vi "RT Loop - Analyze Acceleration_queue_1.vi"(7 "testing":bool, 8 "error in (no error)":errorcluster, 9 "Acceleration RT FIFO In":T1, 10 "FPGA VI Reference Out":refnum<k20>, 11 "Message Queue":refnum<queue>) -> (1 "Acceleration RT FIFO Out":T1)   [LabVIEW 2017]
doc: "Read and analyze acceleration waveform data from FPGA via DMA FIFO. If the acceleration is over the limit, then send the acceleration waveform data to the Log Data Loop."
uses:
  <vilib>/rvi/interface/nirviMethod/nirviMethod.xnode
  <vilib>/FPGAPlugInAG/Dynamic/niLvFpga_ReadFifo_Dynamic.vi
  <vilib>/rvi/errors/niLvFpgaMergeErrorWithErrorCode.vi
  Globals/Global - All RT Loop Stop.vi
  Globals/Global - Configuration Options.vi
  UI Error Handlers/support/Logging/Logging.lvlib
  UI Error Handlers/support/Message Queue/Message Cluster.ctl
  UI Error Handlers/support/Message Queue/Message Queue.lvlib
  controls/Acceleration RT FIFO Reference.ctl
panel:
  out "AVI Path 2":path
  out "G1 status.G1 trigger 3":bool
  out "error out 3":errorcluster
  out "error out 2":errorcluster
  out "AVI Path":path
  out "G1 status.G1 trigger 2":bool
  out "error out":errorcluster
  out "Array":waveform(dbl)[](array[waveform])
  out "x-y":u32
  out "G1 status":cluster{"G1 trigger":bool}
  out "G1 status.G1 trigger":bool
  out "sta":bool
  out "logical OR":bool
  in  "Data Rate (Hz)":dbl
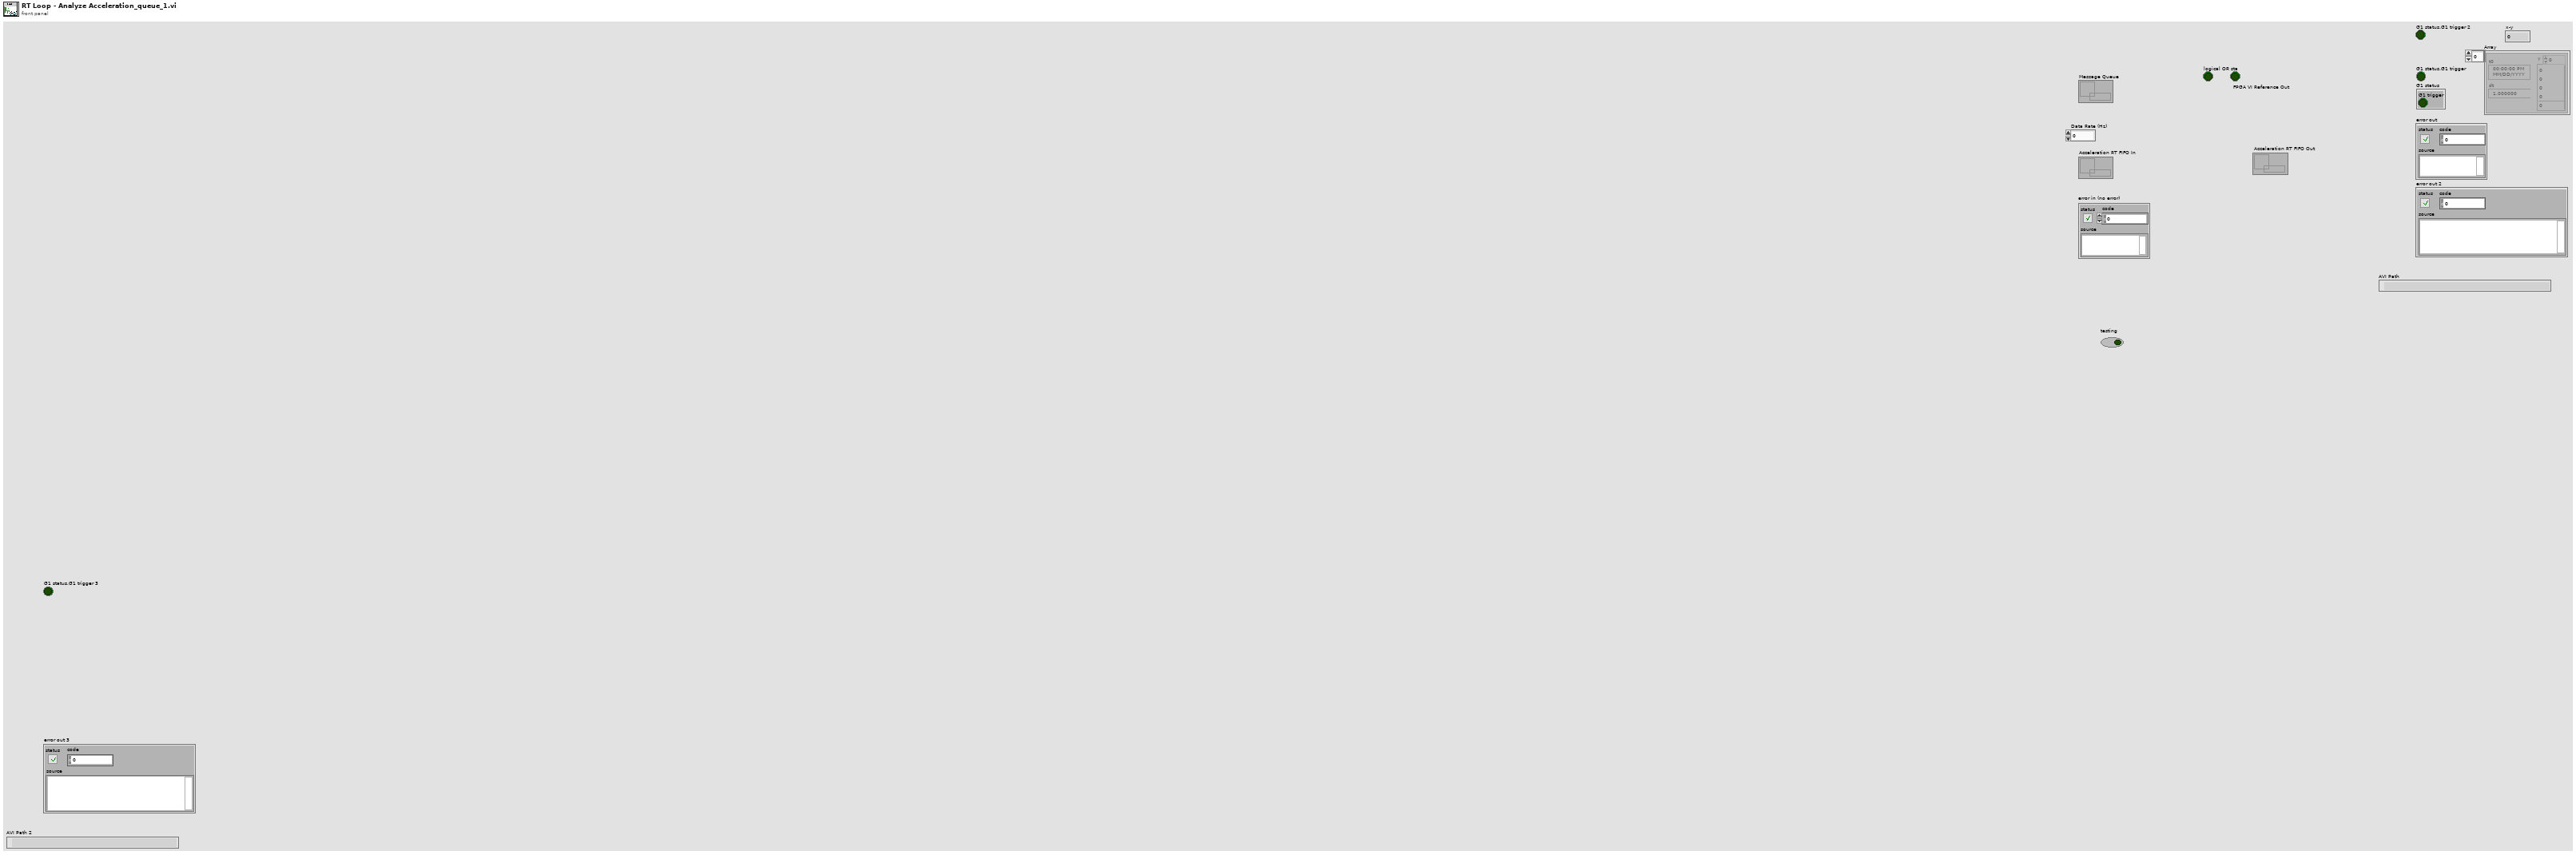
[diagram p1: front panel]
types:
  T1 = typedef "Acceleration RT FIFO Reference.ctl" = refnum<k33>
  T2 = cluster{"Tool data":cluster{"Number of teeth":sgl}, "Cutting data":cluster{"rpm":sgl}, "Limits":cluster{"Magnitude threshold":sgl, "Tolerance":sgl}, "G1 status":cluster{"G1 trigger":bool}}
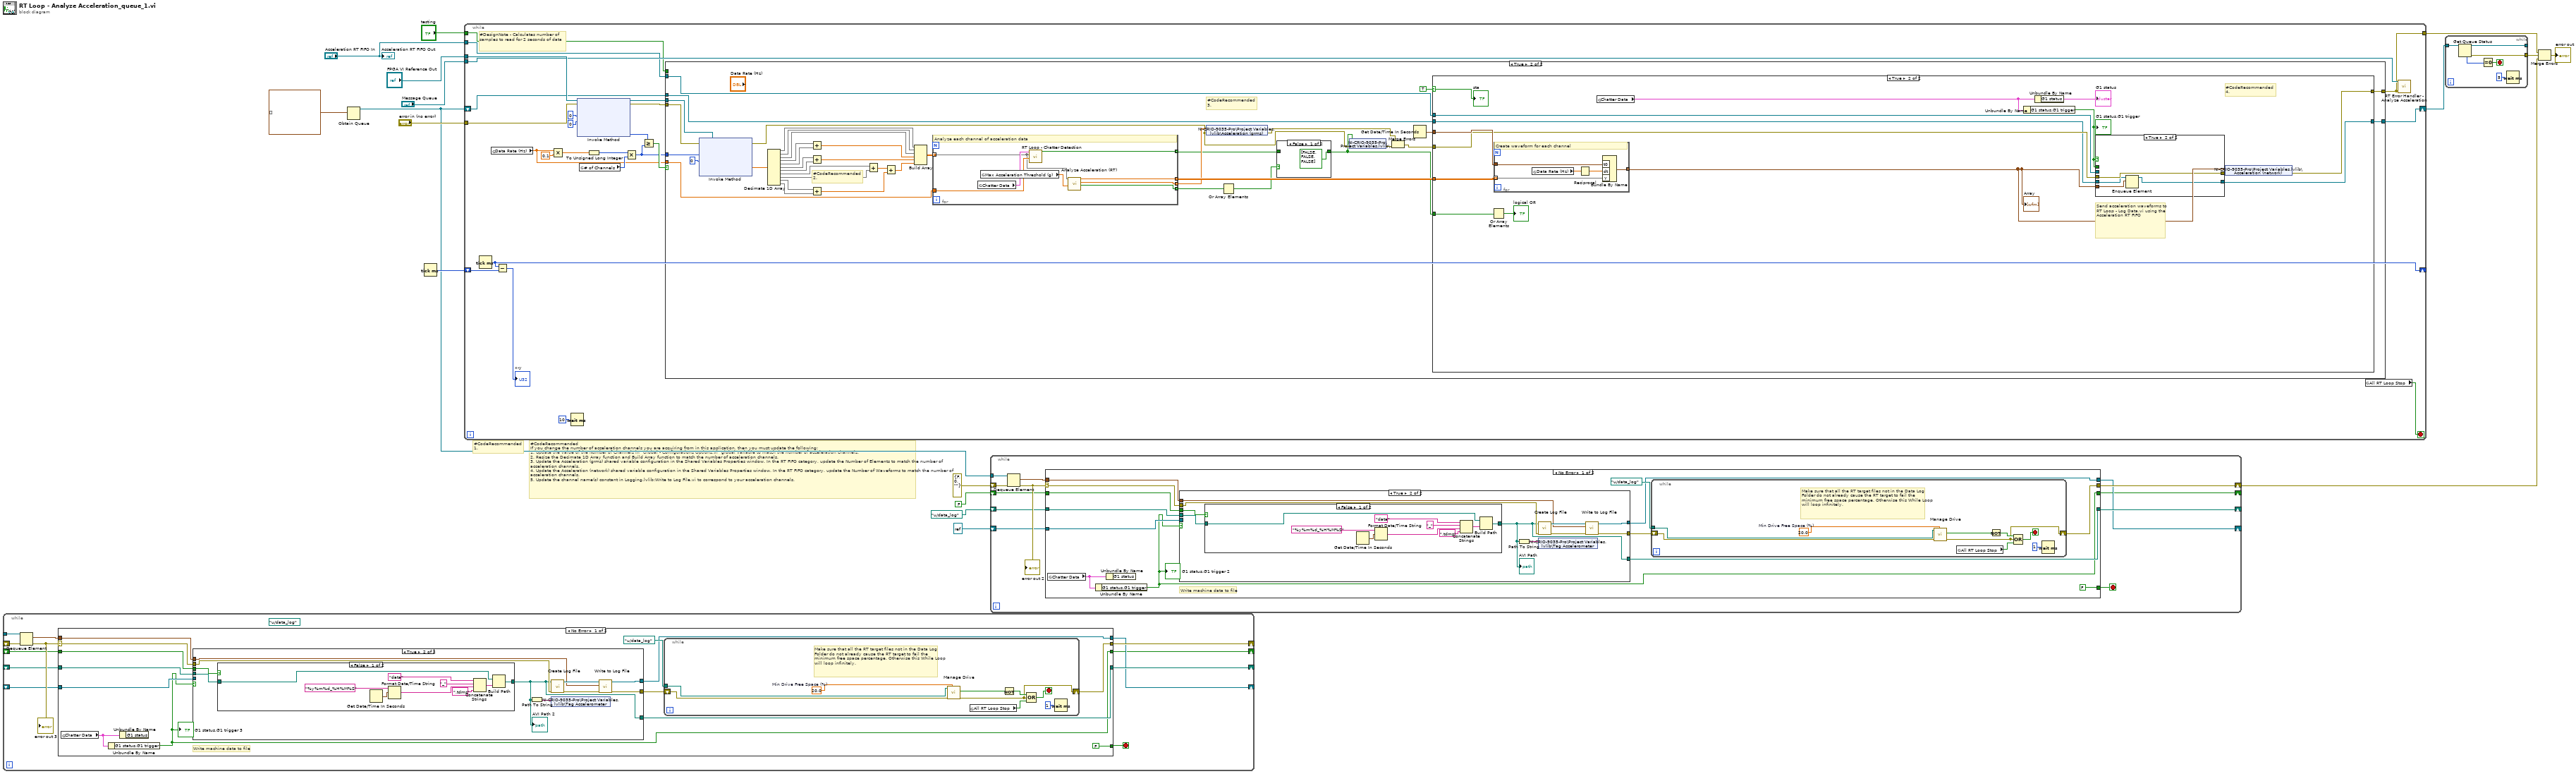
[diagram p0: block diagram]
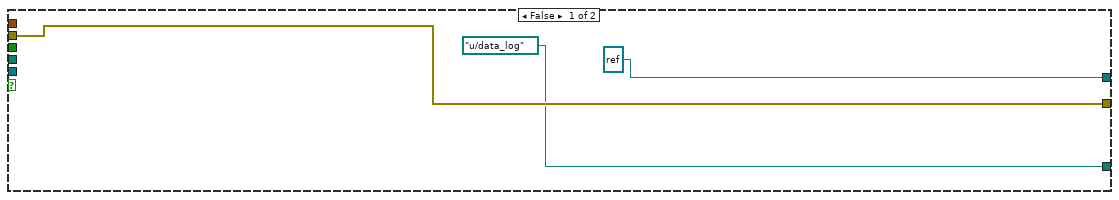
[diagram p2: hidden frame]
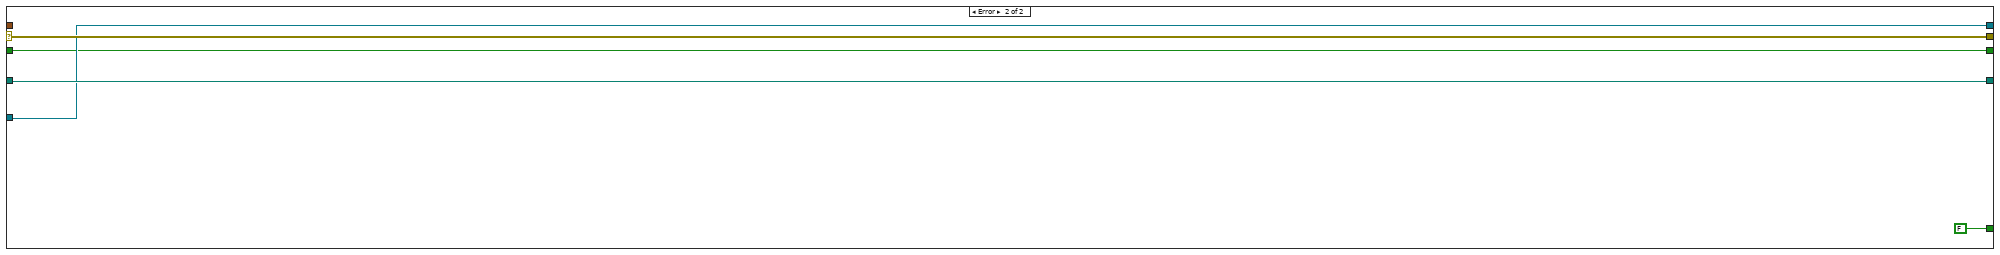
[diagram p4: hidden frame]
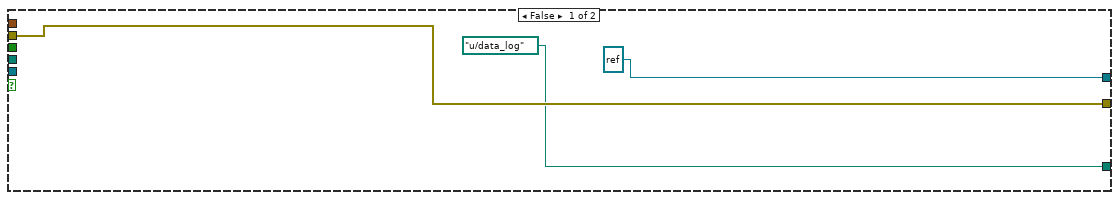
[diagram p5: hidden frame]
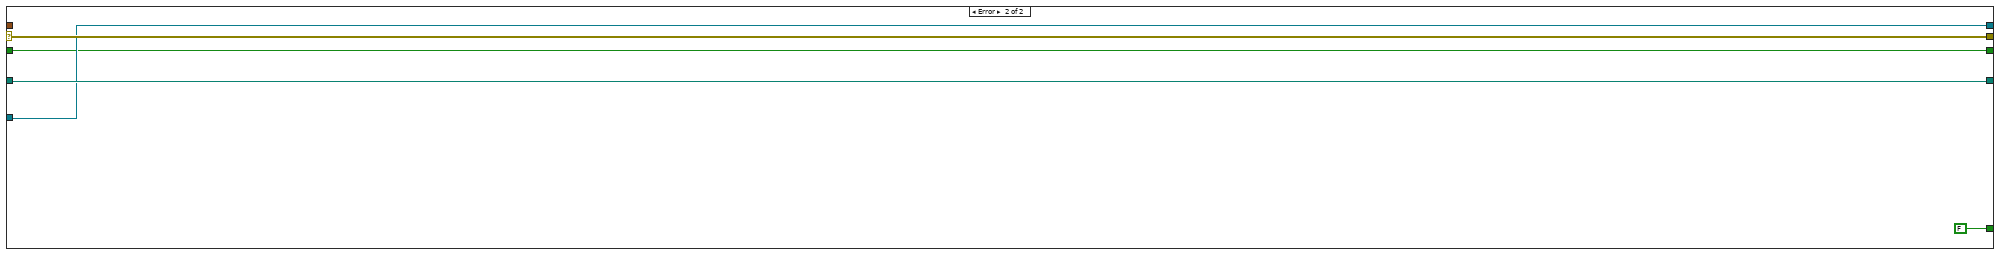
[diagram p7: hidden frame]
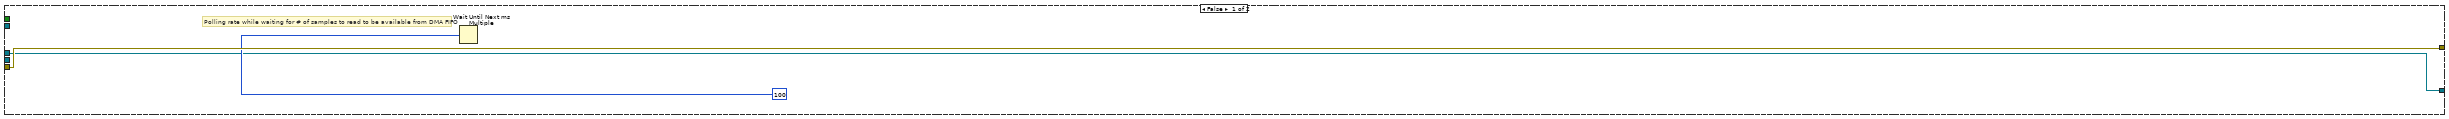
[diagram p8: hidden frame]
diagram:
  (unwired) path "u:/data_log" ("AVI Path")
  # "#CodeRecommended\n1."
  # "#CodeRecommended\nIf you change the number of acceleration channels you are acquiring from in this application, then you must update the following:\n1. Update the value of the Number of Channels in \"Global - Configurations Options.vi\" global variable to match the number of acceleration channels.\n2. Resize the Decimate 1D Array function and Build Array function to match the number of acceleration channels. \n3. Update the Acceleration (grms) shared variable configuration in the Shared Variables Properties window. In the RT FIFO category, update the Number of Elements to match the number of acceleration channels. \n4. Update the Acceleration (network) shared variable configuration in the Shared Variables Properties window. In the RT FIFO category, update the Number of Waveforms to match the number of acceleration channels.\n5. Update the channel name(s) constant in Logging.lvlib:Write to Log File.vi to correspond to your acceleration channels."
  n1 = while {
    tunnel: _ -> [w29]
    shift-right: [w25] -> _
    shift-left: _ -> [w28]
    shift-right: [w18] -> _
    shift-left: _ -> [w21]
    shift-right: [w23] -> _
    shift-left: _ -> [w24]
    shift-right: [w20] -> _
    shift-left: _ -> [w19]
    stop <- w26 stop-if-true
    n2 = Dequeue Element(queue=w29, error in (no error)=w28) -> (element=w22:waveform(dbl)[], error out=w27:errorcluster)  [unwired: 1 in, 2 out]
    "error out 3" <- w27
    n3 = case shown="No Error" w27 {
      selector: w27 -> [w37 w78]
      tunnel: [FALSE FALSE] -> w26
      tunnel: [w35 w78] -> w25
      tunnel: w24 -> [w41 w77]
      tunnel: [w40 w77] -> w23
      tunnel: w22 -> [w39 _]
      tunnel: w21 -> [w34 w75]
      tunnel: [w33 w76] -> w20
      tunnel: w19 -> [w32 w76]
      tunnel: [w30 w75] -> w18
      frame No Error {
        # "Write machine data to file"
        n4 = global read "Global - Configuration Options.vi" "Chatter Data"() -> (w31:T2)
        n5 = Unbundle By Name(w31) -> ("G1 status.G1 trigger"=w30:bool)
        "G1 status.G1 trigger 3" <- w30
        n6 = Unbundle By Name(w31) -> ()  [unwired: 1 out]
        n7 = case shown="True" w30 {
          tunnel: w41 -> [_ w64]
          tunnel: [path "u:/data_log" ("AVI Path") w56] -> w40
          tunnel: w39 -> [_ w60]
          tunnel: w37 -> [w54 w59]
          tunnel: [w54 w58] -> w36
          tunnel: w34 -> [_ w55]
          tunnel: [refnum<k34> refnum ("Log File out") w57] -> w33
          tunnel: w32 -> [_ _]
          frame False {
          }
          frame True {
            n8 = case shown="False" w55 {
              tunnel: w64 -> [w67 w74]
              tunnel: [w66 w74] -> w56
              frame False {
                n9 = Get Date/Time In Seconds() -> (seconds since 1Jan1904=w69:timestamp)
                n10 = Format Date/Time String(time format string (%c)="%y%m%d_%H%M%S", seconds (now)=w69) -> (date/time string=w72:string)  [unwired: 1 out]
                n11 = Concatenate Strings("data" ("string"), "_" ("string"), w72, ".tdms" ("string")) -> (w68:string)
                n12 = Build Path(base path=w67, name or relative path=w68) -> (appended path=w66:path)
              }
              frame True {
              }
            }
            "AVI Path 2" <- w56
            n13 = Path To String(path=w56) -> (string=w61:string)
            n14 = call "Create Log File.vi"("error in (no error)"=w59, "Acceleration Exceeded Log Folder"=w56) -> ("error out"=w63:errorcluster, "Log File out"=w62:refnum<k34>)  [unwired: 8 in]
            n15 = shared-variable "NI-CRIO-9035-Pro\\Project Variables.lvlib\\Tag Accelerometer"(w61) -> ()  [unwired: 1 in, 1 out]
            n16 = call "Write to Log File.vi"("error in (no error)"=w63, "Array of Waveforms"=w60, "Log File in"=w62) -> ("error out"=w58:errorcluster, "Log File out"=w57:refnum<k34>)  [unwired: 7 in]
          }
        }
        n17 = while {
          shift-right: [w46] -> w35
          shift-left: w36 -> [w47]
          tunnel: path "u:/data_log" ("AVI Path") -> [w44]
          stop <- w51 stop-if-true
          w45 = 20.0  # Min Drive Free Space (%)
          # "Make sure that all the RT target files not in the Data Log Folder do not already cause the RT target to fail the minimum free space percentage. Otherwise this While Loop will loop infinitely."
          n18 = call "Manage Drive.vi"("Min Drive Free Space (%)"=w45, "error in"=w47, "Data Folder"=w44) -> ("error out"=w46:errorcluster, "Drive Space Below Limit"=w43:bool)  [unwired: 7 in]
          n19 = global read "Global - All RT Loop Stop.vi" "All RT Loop Stop"() -> (w48:bool)
          n20 = Not(x=w43) -> (.not. x?=w50:bool)
          n21 = Compound Arithmetic op=OR(w50, w46, w48) -> (w51:bool)
          n22 = Wait (ms)(milliseconds to wait=u32 1) -> ()  [unwired: 1 out]
        }
      }
      frame Error {
      }
    }
  }
  n23 = Obtain Queue(element data type=waveform(dbl)[] [] ("Array 2")) -> (queue out=w5:refnum<queue>)  [unwired: 4 in, 2 out]
  n24 = Tick Count (ms)() -> (millisecond timer value=w12:u32)
  n25 = while {
    tunnel: "FPGA VI Reference Out" -> [w104]
    tunnel: "error in (no error)" -> [w103]
    tunnel: "Message Queue" -> [w96]
    tunnel: "Acceleration RT FIFO In" -> [w95]
    tunnel: "testing" -> [w87]
    shift-right: [w85] -> _
    shift-left: w12 -> [w86]
    shift-right: [w82] -> w4
    shift-left: w5 -> [w83]
    tunnel: [w81] -> w2
    stop <- w97 stop-if-true
    # "#DesignNote - Calculates number of samples to read for 2 seconds of data"
    n26 = Tick Count (ms)() -> (millisecond timer value=w85:u32)
    n27 = global read "Global - Configuration Options.vi" "Data Rate (Hz)"() -> (w89:dbl)
    n28 = Subtract(x=w85, y=w86) -> (x-y=→"x-y":u32)
    n29 = Multiply(x=w89, y=0.1) -> (x*y=w93:dbl)
    n30 = Wait (ms)(milliseconds to wait=u32 10) -> ()  [unwired: 1 out]
    n31 = xnode "Invoke Method"("FPGA VI Reference In"=w104, "error in"=w103, "Number of Elements"=u32 0, "Timeout (ms)"=0) -> ("FPGA VI Reference Out"=w100:refnum<k20>, "error out"=w99:errorcluster, "Elements Remaining"=w88:u32)  [unwired: 1 out]
    n32 = global read "Global - Configuration Options.vi" "# of Channels"() -> (w90:u32)
    n33 = To Unsigned Long Integer(number=w93) -> (unsigned 32bit integer=w92:u32)
    n34 = Multiply(x=w92, y=w90) -> (x*y=w91:u32)
    n35 = Greater Or Equal?(x=w88, y=w91) -> (x >= y?=w98:bool)
    n36 = case shown="True" w98 {
      tunnel: w100 -> [_ w146]
      tunnel: w99 -> [w107 w145]
      tunnel: [w107 w141] -> w81
      tunnel: w91 -> [_ w144]
      tunnel: w95 -> [_ w139]
      tunnel: w89 -> [_ w135]
      tunnel: w87 -> [_ _]
      tunnel: w83 -> [w105 w109]
      tunnel: [w105 w108] -> w82
      frame False {
        # "Polling rate while waiting for # of samples to read to be available from DMA FIFO"
        n37 = Wait Until Next ms Multiple(millisecond multiple=u32 100) -> ()  [unwired: 1 out]
      }
      frame True {
        # "#CodeRecommended\n3."
        # "#CodeRecommended\n2."
        n38 = xnode "Invoke Method"("FPGA VI Reference In"=w146, "error in"=w145, "Number of Elements"=w144, "Timeout (ms)"=0) -> ("error out"=w134:errorcluster, "Data"=w138:sgl[])  [unwired: 2 out]
        n39 = Decimate 1D Array(w138) -> (w125:sgl[], w124:sgl[], w123:sgl[], w122:sgl[], w121:sgl[], w119:sgl[], w118:sgl[], w117:sgl[], w116:sgl[], w115:sgl[], w114:sgl[])
        n40 = Add(x=w122, y=w121) -> (x+y=w120:sgl[])
        n41 = Add(x=w119, y=w118) -> (x+y=w110:sgl[])
        n42 = Add(x=w115, y=w114) -> (x+y=w112:sgl[])
        n43 = Add(x=w117, y=w116) -> (x+y=w113:sgl[])
        n44 = Add(x=w113, y=w112) -> (x+y=w111:sgl[])
        n45 = Build Array(w125, w124, w123, w120, w110, w111) -> (w126:sgl[][])
        n46 = for {
          tunnel: [w156] -> w140 mode=indexing
          tunnel: [w155] -> w137 mode=indexing
          tunnel: [w154] -> w136 mode=indexing
          tunnel: w135 -> [w152]
          tunnel: [w151] -> w129 mode=indexing
          tunnel: w126 -> [w149] mode=indexing
          # "Analyze each channel of acceleration data"
          n47 = global read "Global - Configuration Options.vi" "Chatter Data"() -> (w150:T2)
          n48 = global read "Global - Configuration Options.vi" "Max Acceleration Threshold (g)"() -> (w153:sgl)
          n49 = call "RT Loop - Chatter Detection.vi"("Data Rate (Hz)"=w152, "Acceleration Waveform (SGL)"=w149, "Chatter Data"=w150) -> ("Chatter?"=w151:bool)  [unwired: 8 in]
          n50 = call "Analyze Acceleration (RT).vi"("Max Instantaneous Acceleration (g)"=w153, "Acceleration Waveform (SGL)"=w149) -> ("Over Limit?"=w156:bool, "Acceleration (grms)"=w154:dbl, "Acceleration Waveform (DBL)"=w155:dbl[])  [unwired: 7 in]
        }
        n51 = shared-variable "NI-CRIO-9035-Pro\\Project Variables.lvlib\\Acceleration (grms)"(w136, error in=w134) -> (error out=w132:errorcluster)
        n52 = Or Array Elements(Boolean array=w140) -> (logical OR=w130:bool)
        n53 = case shown="False" w130 {
          tunnel: w129 -> [_ w148]
          tunnel: [bool[] [FALSE, FALSE, FALSE] ("Chatter?") w148] -> w128
          frame False {
          }
          frame True {
          }
        }
        n54 = shared-variable "NI-CRIO-9035-Pro\\Project Variables.lvlib\\Chatter?"(w128, error in=w134) -> (error out=w133:errorcluster)
        n55 = Merge Errors(w132, w133) -> (w131:errorcluster)
        n56 = Get Date/Time In Seconds() -> (seconds since 1Jan1904=w142:timestamp)
        n57 = case shown="True" TRUE {
          selector: TRUE -> [_ w166]
          tunnel: w142 -> [_ w173]
          tunnel: w131 -> [w158 w172]
          tunnel: [w158 w171] -> w141
          tunnel: w139 -> [_ w170]
          tunnel: w137 -> [_ w169]
          tunnel: w128 -> [_ w167]
          tunnel: w109 -> [w157 w160]
          tunnel: [w157 w159] -> w108
          frame False {
          }
          frame True {
            # "#CodeRecommended\n4."
            # "Send acceleration waveforms to RT Loop - Log Data.vi using the Acceleration RT FIFO"
            n58 = Or Array Elements(Boolean array=w167) -> (logical OR=→"logical OR":bool)
            n59 = for {
              tunnel: w169 -> [w184] mode=indexing
              tunnel: w173 -> [w183]
              tunnel: [w181] -> w161 mode=indexing
              # "Create waveform for each channel"
              n60 = global read "Global - Configuration Options.vi" "Data Rate (Hz)"() -> (w180:dbl)
              n61 = Reciprocal(x=w180) -> (1/x=w182:dbl)
              n62 = Bundle By Name("t0"=w183, "dt"=w182, "Y"=w184) -> (w181:waveform(dbl))  [unwired: 1 in]
            }
            "Array" <- w161
            n63 = global read "Global - Configuration Options.vi" "Chatter Data"() -> (w165:T2)
            n64 = Unbundle By Name(w165) -> ("G1 status.G1 trigger"=w162:bool)
            "G1 status.G1 trigger" <- w162
            n65 = Unbundle By Name(w165) -> ("G1 status"=→"G1 status":cluster{"G1 trigger":bool})
            n66 = case shown="True" w162 {
              tunnel: w172 -> [w175 w179]
              tunnel: w161 -> [_ w176]
              tunnel: w170 -> [_ _]
              tunnel: w162 -> [_ _]
              tunnel: [w175 w179] -> w163
              tunnel: w160 -> [w174 w178]
              tunnel: [w174 w177] -> w159
              frame False {
              }
              frame True {
                n67 = Enqueue Element(queue=w178, element=w176) -> (queue out=w177:refnum<queue>)  [unwired: 2 in, 2 out]
              }
            }
            n68 = shared-variable "NI-CRIO-9035-Pro\\Project Variables.lvlib\\Acceleration (network)"(w161, error in=w163) -> (error out=w171:errorcluster)
            "sta" <- w166
          }
        }
      }
    }
    n69 = global read "Global - All RT Loop Stop.vi" "All RT Loop Stop"() -> (w97:bool)
    n70 = call "RT Error Handler - Analyze Acceleration.vi"("error in (no error)"=w81, "Message Queue"=w96) -> ()  [unwired: 9 in, 1 out]
  }
  n71 = while {
    tunnel: w5 -> [w196]
    shift-right: [w192] -> w8
    shift-left: errorcluster {"status"=FALSE, "code"=0, "source"=""} ("error in (no error)") -> [w195]
    shift-right: [w185] -> _
    shift-left: FALSE ("Boolean") -> [w188]
    shift-right: [w190] -> _
    shift-left: path "u:/data_log" ("AVI Path") -> [w191]
    shift-right: [w187] -> _
    shift-left: refnum<k34> refnum ("Log File out") -> [w186]
    stop <- w193 stop-if-true
    n72 = Dequeue Element(queue=w196, error in (no error)=w195) -> (element=w189:waveform(dbl)[], error out=w194:errorcluster)  [unwired: 1 in, 2 out]
    "error out 2" <- w194
    n73 = case shown="No Error" w194 {
      selector: w194 -> [w204 w245]
      tunnel: [FALSE FALSE] -> w193
      tunnel: [w202 w245] -> w192
      tunnel: w191 -> [w208 w244]
      tunnel: [w207 w244] -> w190
      tunnel: w189 -> [w206 _]
      tunnel: w188 -> [w201 w242]
      tunnel: [w200 w243] -> w187
      tunnel: w186 -> [w199 w243]
      tunnel: [w197 w242] -> w185
      frame No Error {
        # "Write machine data to file"
        n74 = global read "Global - Configuration Options.vi" "Chatter Data"() -> (w198:T2)
        n75 = Unbundle By Name(w198) -> ("G1 status.G1 trigger"=w197:bool)
        "G1 status.G1 trigger 2" <- w197
        n76 = Unbundle By Name(w198) -> ()  [unwired: 1 out]
        n77 = case shown="True" w197 {
          tunnel: w208 -> [_ w231]
          tunnel: [path "u:/data_log" ("AVI Path") w223] -> w207
          tunnel: w206 -> [_ w227]
          tunnel: w204 -> [w221 w226]
          tunnel: [w221 w225] -> w203
          tunnel: w201 -> [_ w222]
          tunnel: [refnum<k34> refnum ("Log File out") w224] -> w200
          tunnel: w199 -> [_ _]
          frame False {
          }
          frame True {
            n78 = case shown="False" w222 {
              tunnel: w231 -> [w234 w241]
              tunnel: [w233 w241] -> w223
              frame False {
                n79 = Get Date/Time In Seconds() -> (seconds since 1Jan1904=w236:timestamp)
                n80 = Format Date/Time String(time format string (%c)="%y%m%d_%H%M%S", seconds (now)=w236) -> (date/time string=w239:string)  [unwired: 1 out]
                n81 = Concatenate Strings("data" ("string"), "_" ("string"), w239, ".tdms" ("string")) -> (w235:string)
                n82 = Build Path(base path=w234, name or relative path=w235) -> (appended path=w233:path)
              }
              frame True {
              }
            }
            "AVI Path" <- w223
            n83 = Path To String(path=w223) -> (string=w228:string)
            n84 = call "Create Log File.vi"("error in (no error)"=w226, "Acceleration Exceeded Log Folder"=w223) -> ("error out"=w230:errorcluster, "Log File out"=w229:refnum<k34>)  [unwired: 8 in]
            n85 = shared-variable "NI-CRIO-9035-Pro\\Project Variables.lvlib\\Tag Accelerometer"(w228) -> ()  [unwired: 1 in, 1 out]
            n86 = call "Write to Log File.vi"("error in (no error)"=w230, "Array of Waveforms"=w227, "Log File in"=w229) -> ("error out"=w225:errorcluster, "Log File out"=w224:refnum<k34>)  [unwired: 7 in]
          }
        }
        n87 = while {
          shift-right: [w213] -> w202
          shift-left: w203 -> [w214]
          tunnel: path "u:/data_log" ("AVI Path") -> [w211]
          stop <- w218 stop-if-true
          w212 = 20.0  # Min Drive Free Space (%)
          # "Make sure that all the RT target files not in the Data Log Folder do not already cause the RT target to fail the minimum free space percentage. Otherwise this While Loop will loop infinitely."
          n88 = call "Manage Drive.vi"("Min Drive Free Space (%)"=w212, "error in"=w214, "Data Folder"=w211) -> ("error out"=w213:errorcluster, "Drive Space Below Limit"=w210:bool)  [unwired: 7 in]
          n89 = global read "Global - All RT Loop Stop.vi" "All RT Loop Stop"() -> (w215:bool)
          n90 = Not(x=w210) -> (.not. x?=w217:bool)
          n91 = Compound Arithmetic op=OR(w217, w213, w215) -> (w218:bool)
          n92 = Wait (ms)(milliseconds to wait=u32 1) -> ()  [unwired: 1 out]
        }
      }
      frame Error {
      }
    }
  }
  n93 = while {
    tunnel: [w251] -> w3
    tunnel: [w249] -> _
    tunnel: w4 -> [w247]
    stop <- w250 stop-if-true
    n94 = Get Queue Status(queue=w247) -> (queue out=w249:refnum<queue>, error out=w251:errorcluster, # elements in queue=w248:i32)  [unwired: 2 in, 5 out]
    n95 = Equal To 0?(x=w248) -> (x = 0?=w250:bool)
    n96 = Wait (ms)(milliseconds to wait=u32 5) -> ()  [unwired: 1 out]
  }
  n97 = Merge Errors(w2, w3, w8) -> (→"error out":errorcluster)
  "Acceleration RT FIFO Out" <- "Acceleration RT FIFO In"
